vi "Run Runnable.vi"(8 "error in (no error)":errorcluster, 10 "Runnable":refnum<class "Runnable.lvclass">, 11 "Parallell Test Runner In":refnum<class "Parallell Test Runner.lvclass">) -> (0 "error out":errorcluster, 3 "Parallell Test Runner Out":refnum<class "Parallell Test Runner.lvclass">)   [LabVIEW 2020, in "Parallell Test Runner.lvclass"]
uses:
  Parallell Test Runner.lvclass
  Core/Runnable/Runnable.lvclass
  Parallell Test Runner.lvclass/Parallell Test Runner.ctl
  Private/Runner.vi
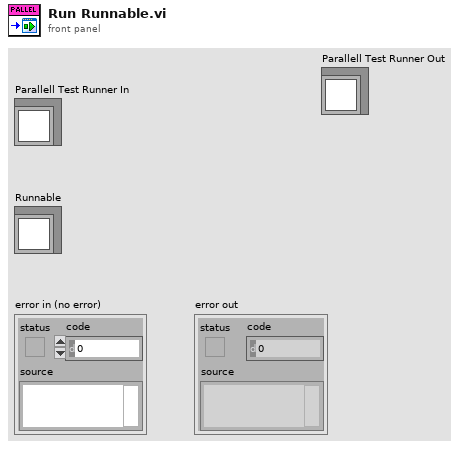
[diagram p1: front panel]
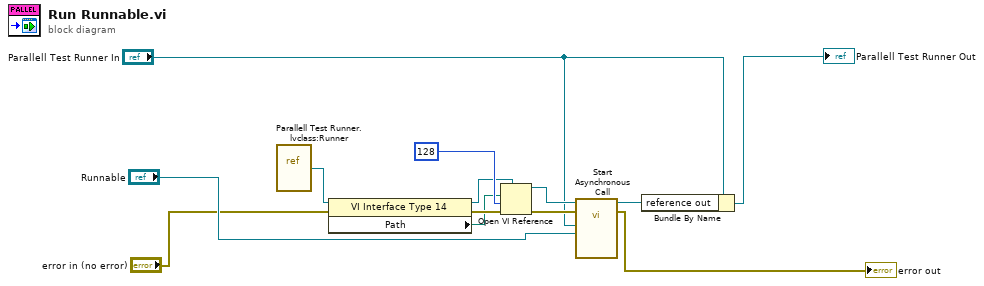
[diagram p0: block diagram]
diagram:
  n1 = vi-ref "Parallell Test Runner.lvclass:Runner.vi"() -> (w7:refnum<vi>)
  n2 = property class="VI Interface Type 14"(reference=w7, error in="error in (no error)") -> (reference out=w9:refnum<vi>, error out=w10:errorcluster, "Path"=w8:path)
  n3 = Open VI Reference(type specifier VI Refnum (for type only)=w9, vi path=w8, options=128, error in (no error)=w10) -> (vi reference=w11:refnum<vi>, error out=w12:errorcluster)  [unwired: 2 in]
  n4 = call-by-ref "Start Asynchronous Call"(reference=w11, error in=w12, "Runnable"="Runnable", "Parallell Test Runner In"="Parallell Test Runner In") -> (reference out=w1:refnum<vi>, error out=→"error out":errorcluster)  [unwired: 9 in, 1 out]
  n5 = Bundle By Name(cluster="Parallell Test Runner In", "reference out"=w1) -> (→"Parallell Test Runner Out":refnum<class "Parallell Test Runner.lvclass">)
